vi "Initialize TDK 20-38.vi"(8 "error in (no error)":errorcluster, 11 "Device position":string) -> (0 "error out":errorcluster, 3 "VISA out":refnum<visa-resource-name>)   [LabVIEW 2023, in "TDK20-38 API.lvlib"]
uses:
  TDK20-38 API.lvlib
  <userlib>/TDK-Lambda GEN LAN Series/TDK-Lambda GEN LAN Series.lvlib
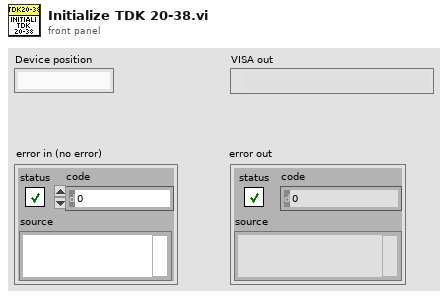
[diagram p1: front panel]
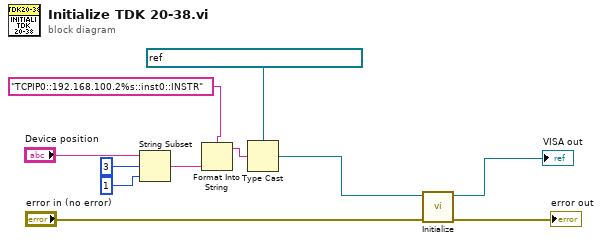
[diagram p0: block diagram]
diagram:
  n1 = String Subset(string="Device position", offset (0)=3, length (rest)=1 ("length (rest)")) -> (substring=w4:string)
  n2 = Format Into String(format string="TCPIP0::192.168.100.2%s::inst0::INSTR" ("Adress"), w4) -> (resulting string=w2:string)  [unwired: 2 in, 1 out]
  n3 = Type Cast(type=refnum<visa-resource-name> "TCPIP0::192.168.100.21::inst0::INSTR" ("VISA name"), x=w2) -> (*(type *) &x=w9:refnum<visa-resource-name>)
  n4 = call "Initialize.vi"("error in (no error)"="error in (no error)", "VISA name"=w9) -> ("error out"=→"error out":errorcluster, "VISA out"=→"VISA out":refnum<visa-resource-name>)  [unwired: 8 in]
